vi "Image_processor.vi"(6 "DUT":u16, 9 "Ref Folder":path, 10 "DUT_Conf":string="RX-DUT", 11 "Image Path":path) -> (2 "Fail_Strings":string, 3 "PASS/FAIL":bool)   [LabVIEW 2025]
uses:
  Image_match_details.ctl
  <vilib>/Utility/file.llb/Read Delimited Spreadsheet (string).vi
panel:
  out "Array 3":T1[](array[typedef])
  out "Array 2":T1[](array[typedef])
  out "DUT":T2(plugin-control)
  out "Array":i32[](array[numeric])
  # "RY-DUT"
  # "RX-DUT"
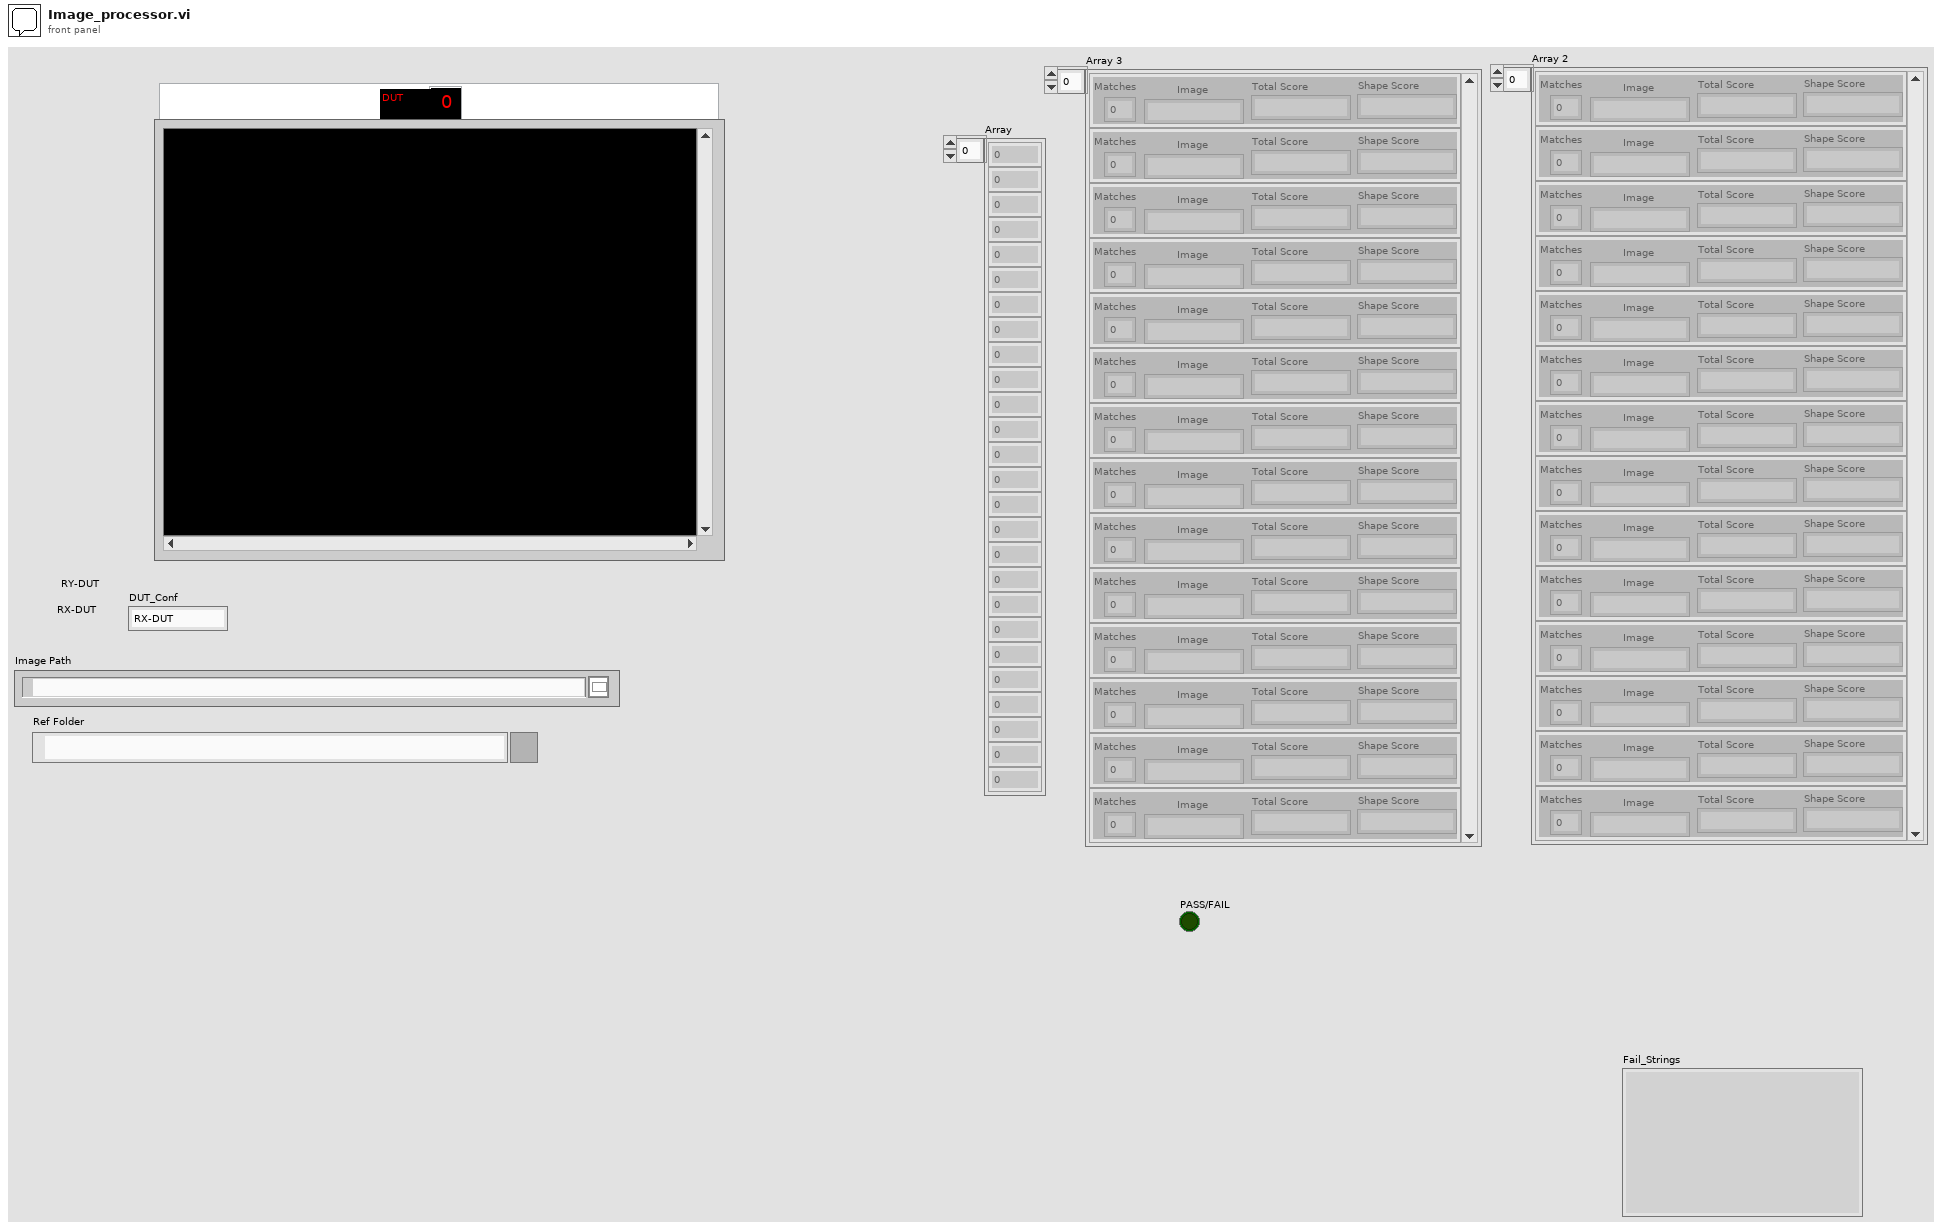
[diagram p1: front panel]
types:
  T1 = typedef "Image_match_details.ctl" = cluster{"Matches":i32, "Image":string, "Total Score":string, "Shape Score":string}
  T2 = typedef "IMAQ Image.ctl" = refnum<image>
  T3 = typedef "Image Type" = u32
  T4 = enum16{"open", "replace", "create", "open or create", "replace or create", "replace or create with confirmation"}
  T5 = cluster{"Position":cluster{"x":sgl, "y":sgl}, "Angle":sgl, "Scale":sgl, "Score":sgl, "Bounding Box":cluster{"x":sgl, "y":sgl}[]}
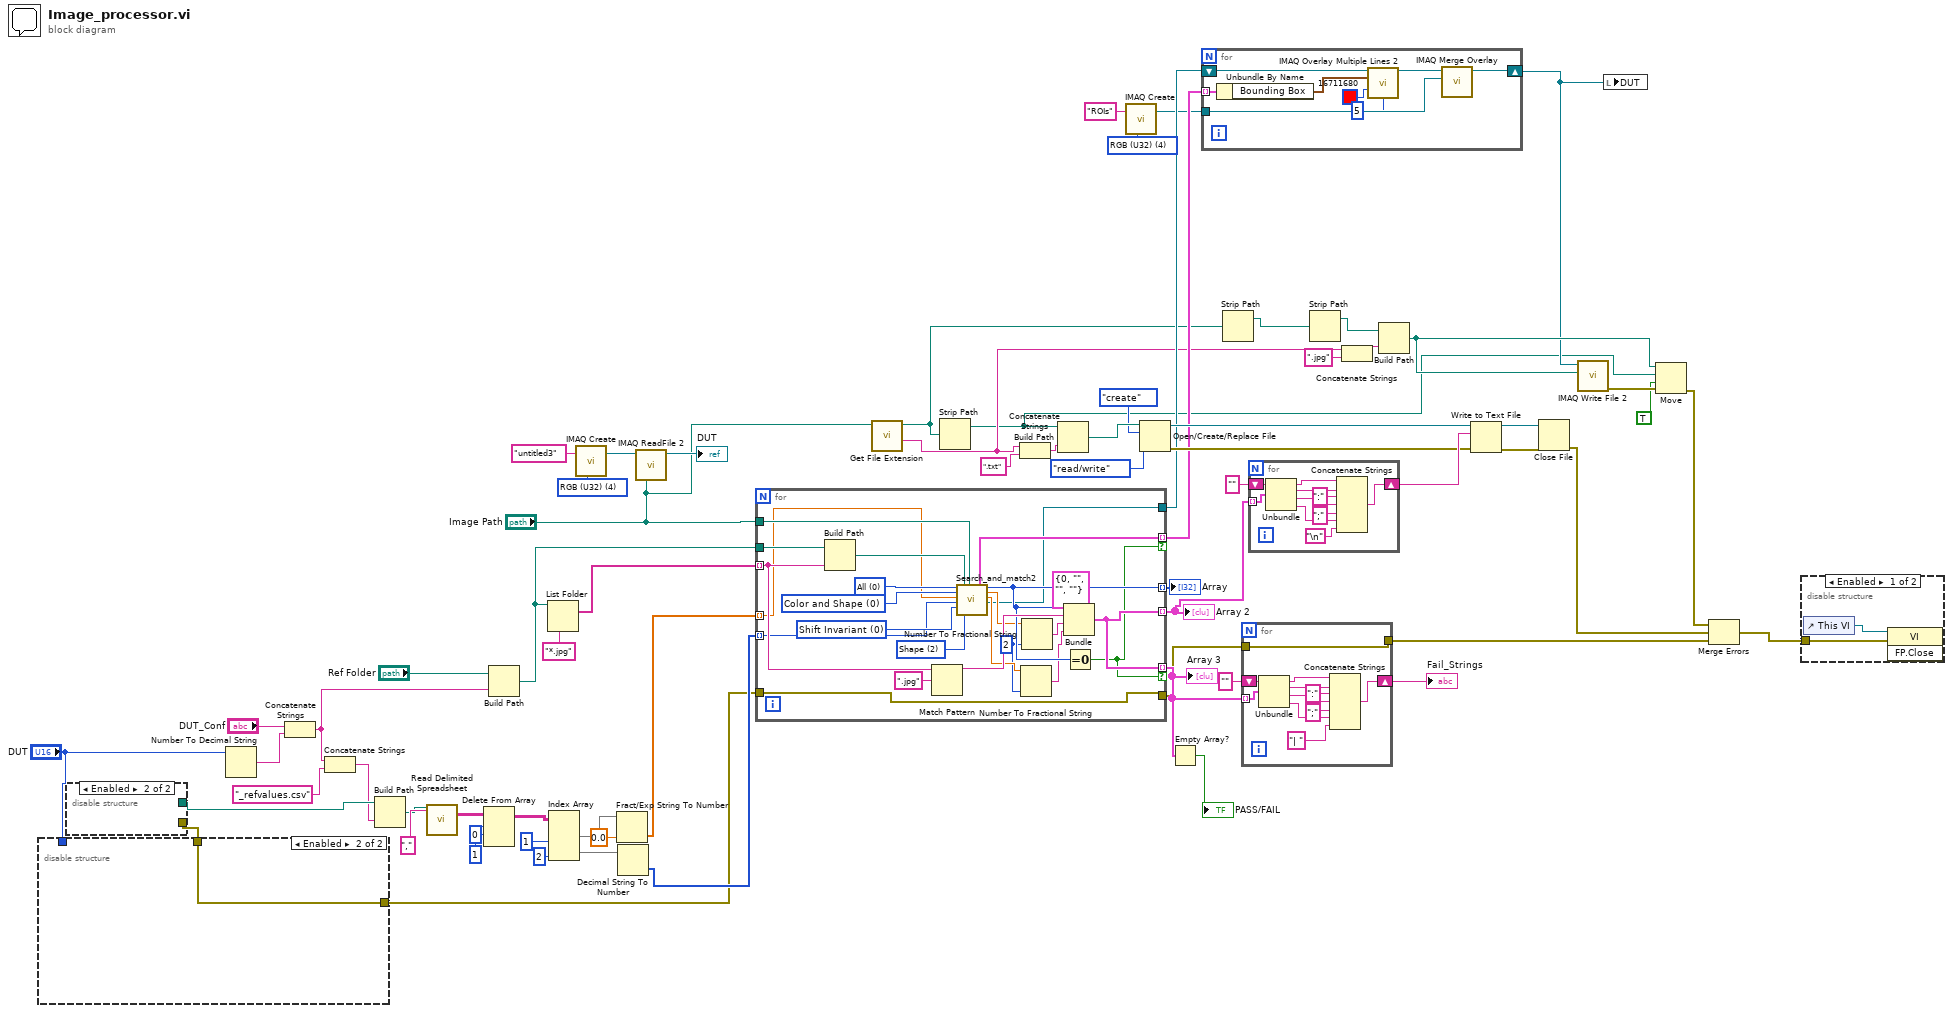
[diagram p0: block diagram]
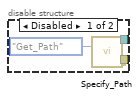
[diagram p2: hidden frame]
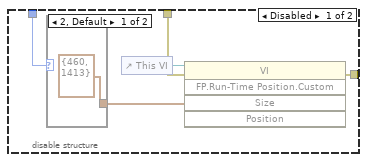
[diagram p3: hidden frame]
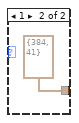
[diagram p4: hidden frame]
diagram:
  w17 = T3 4 items=["Grayscale (U8)", "Grayscale (I16)", "Grayscale (SGL)", "Complex (CSG)", "RGB (U32)", "HSL (U32)", "RGB (U64)", "Grayscale (U16)"] ("Image Type")
  w41 = T3 4 items=["Grayscale (U8)", "Grayscale (I16)", "Grayscale (SGL)", "Complex (CSG)", "RGB (U32)", "HSL (U32)", "RGB (U64)", "Grayscale (U16)"] ("Image Type")
  n1 = disable-structure shown="Enabled" {
    disable-tunnel: [w71 _] -> w51
    disable-tunnel: [w70 _] -> w37
    frame Disabled {
      n2 = call "Specify_Path.vi"("Path_Enum"=enum16{"Find_Path", "Get_Path"}."Get_Path") -> ("Configurations"=w71:path, "error out"=w70:errorcluster)  [unwired: 7 in, 6 out]
    }
    frame Enabled {
    }
  }
  n3 = disable-structure shown="Enabled" {
    disable-tunnel: w37 -> [w76 w80]
    disable-tunnel: "DUT" -> [w75 _]
    disable-tunnel: [w73 w80] -> w35
    frame Disabled {
      n4 = case shown="2, Default" w75 {
        tunnel: [cluster{"Top":i16, "Left":i16} {"Top"=460, "Left"=1413} ("Position") cluster{"Top":i16, "Left":i16} {"Top"=384, "Left"=41} ("Position")] -> w74
        frame 2, Default {
        }
        frame 1 {
        }
      }
      n5 = control-ref of="This VI"() -> (w77:refnum<vi>)
      n6 = invoke class="VI" method="FP.Run-Time Position.Custom"(reference=w77, error in=w76, "Size"=w74) -> (error out=w73:errorcluster)  [unwired: 2 in, 4 out]
    }
    frame Enabled {
    }
  }
  n7 = Number To Decimal String(number="DUT") -> (decimal integer string=w68:string)  [unwired: 1 in]
  n8 = Concatenate Strings("DUT_Conf", w68) -> (w53:string)
  n9 = Concatenate Strings(w53, "_refvalues.csv") -> (w50:string)
  n10 = Build Path(base path=w51, name or relative path=w50) -> (appended path=w49:path)
  n11 = call-poly <vilib>:"Read Delimited Spreadsheet.vi"("file path (dialog if empty)"=w49, "delimiter (\\t)"="," ("delimiter (\\t)")) -> ("all rows"=w61:string[][])  [unwired: 8 in, 5 out]
  n12 = Delete From Array(array=w61, length=1, index (row)=0) -> (array with subset deleted=w56:string[][])  [unwired: 1 in, 1 out]
  n13 = Build Path(base path="Ref Folder", name or relative path=w53) -> (appended path=w65:path)
  n14 = List Folder(path=w65, pattern="*.jpg") -> (filenames=w66:string[])  [unwired: 2 in, 3 out]
  n15 = Index Array(array=w56, index (col) #1=1 ("disabled index (col)"), index (col) #2=2 ("disabled index (col)")) -> (element #1=w58:string[], element #2=w57:string[])  [unwired: 2 in]
  n16 = call "IMAQ Create"("Image Name"="untitled3", "Image Type"=w41) -> ("New Image"=w39:T2)  [unwired: 3 in, 1 out]
  n17 = Fract/Exp String To Number(string=w58, default (0 dbl)=sgl 0.0 ("default (0 DBL)")) -> (number=w48:sgl[])  [unwired: 2 in, 1 out]
  n18 = Decimal String To Number(string=w57) -> (number=w47:i32[])  [unwired: 2 in, 1 out]
  n19 = call "IMAQ ReadFile 2"("File Path"="Image Path", "Image"=w39) -> ("Image Out"=→"DUT":T2)  [unwired: 5 in, 4 out]
  n20 = for {
    tunnel: w66 -> [w97] mode=indexing
    tunnel: w65 -> [w104]
    tunnel: "Image Path" -> [w102]
    tunnel: [w92] -> w64 mode=indexing
    tunnel: [w91] -> w32 mode=indexing
    tunnel: w48 -> [w94] mode=indexing
    tunnel: w47 -> [w93] mode=indexing
    tunnel: [w91] -> w43 mode=indexing if=w81
    tunnel: w35 -> [w88]
    tunnel: [w88] -> w34
    tunnel: [w83] -> w20 mode=indexing if=w81
    tunnel: [w82] -> w19
    w86 = i16 2 ("precision (6)")
    w98 = u32 2 items=["Color and Shape", "Color", "Shape"] ("Match Feature Mode")
    w99 = u32 0 items=["Shift Invariant", "Rotation Invariant"] ("Match Mode")
    w100 = u32 0 items=["Color and Shape", "Color", "Shape "] ("Feature Mode")
    w101 = u32 0 items=["All", "Shift Information", "Rotation Information"] ("Learn Mode")
    n21 = Build Path(base path=w104, name or relative path=w97) -> (appended path=w103:path)
    n22 = Match Pattern(string=w97, regular expression=".jpg") -> (before substring=w95:string)  [unwired: 1 in, 3 out]
    n23 = call "Search_and_match2.vi"("Learn Mode"=w101, "Feature Mode"=w100, "Minimum Match Score"=w94, "Number of Matches Requested"=w93, "Match Mode"=w99, "Ref path"=w103, "Match Feature Mode"=w98, "Main Path"=w102) -> ("Match values"=w83:T5, "Number of Matches"=w92:i32, "Total Score"=w90:sgl, "Shape Score"=w87:sgl, "Main Image"=w82:T2)  [unwired: 7 in]
    n24 = Number To Fractional String(number=w87, precision (6)=w86) -> (F-format string=w85:string)  [unwired: 2 in]
    n25 = Number To Fractional String(number=w90, precision (6)=w86) -> (F-format string=w89:string)  [unwired: 2 in]
    n26 = Bundle(cluster=T1 {"Matches"=0, "Image"="", "Total Score"="", "Shape Score"=""} ("output cluster"), "Matches"=w92, "Image"=w95, "Total Score"=w89, "Shape Score"=w85) -> (w91:T1)
    n27 = Equal To 0?(x=w92) -> (x = 0?=w81:bool)
  }
  "Array" <- w64
  "Array 2" <- w32
  "Array 3" <- w43
  n28 = call <vilib>:"Get File Extension.vi"("file"="Image Path") -> ("filename without extension"=w9:string, "dup file"=w12:path)  [unwired: 6 in, 3 out]
  n29 = Strip Path(path=w12) -> (stripped path=w4:path)  [unwired: 1 out]
  n30 = Concatenate Strings(w9, ".txt" ("string")) -> (w31:string)
  n31 = Build Path(base path=w4, name or relative path=w31) -> (appended path=w29:path)
  n32 = call "IMAQ Create"("Image Name"="ROIs", "Image Type"=w17) -> ("New Image"=w16:T2)  [unwired: 3 in, 1 out]
  n33 = Open/Create/Replace File(file path (use dialog)=w29, operation (0:open)=T4."create", access (0:read/write)=enum16{"read/write", "read-only", "write-only"}."read/write") -> (refnum out=w26:refnum<file>, error out=w25:errorcluster)  [unwired: 3 in, 1 out]
  n34 = Empty Array?(array=w43) -> (empty?=→"PASS/FAIL":bool)
  n35 = for {
    tunnel: w20 -> [w110] mode=indexing
    shift-right: [w107] -> w5
    shift-left: w19 -> [w112]
    tunnel: w16 -> [w106]
    n36 = Unbundle By Name(w110) -> ("Bounding Box"=w109:cluster{"x":sgl, "y":sgl}[])
    n37 = call "IMAQ Overlay Multiple Lines 2"("Image"=w112, "Line End Points"=w109, "Color"=u32 16711680, "Width"=u32 5) -> ("Image Out"=w108:T2)  [unwired: 10 in, 1 out]
    n38 = call "IMAQ Merge Overlay"("Image Dst"=w106, "Image Src"=w108) -> ("Image Dst Out"=w107:T2)  [unwired: 8 in, 1 out]
  }
  n39 = Strip Path(path=w12) -> (stripped path=w3:path)  [unwired: 1 out]
  n40 = for {
    tunnel: w43 -> [w122] mode=indexing
    shift-right: [w117] -> w44
    shift-left: "" -> [w116]
    tunnel: w34 -> [w115]
    tunnel: [w115] -> w33
    n41 = Unbundle(w122) -> ("Image"=w121:string, "Total Score"=w119:string, "Shape Score"=w113:string)  [unwired: 1 out]
    n42 = Concatenate Strings(w116, w121, ":" ("string"), w119, ";" ("string"), w113, "| " ("string")) -> (w117:string)
  }
  "Fail_Strings" <- w44
  n43 = for {
    tunnel: w32 -> [w131] mode=indexing
    shift-right: [w127] -> w27
    shift-left: "" -> [w126]
    n44 = Unbundle(w131) -> ("Image"=w130:string, "Total Score"=w128:string, "Shape Score"=w124:string)  [unwired: 1 out]
    n45 = Concatenate Strings(w126, w130, ":" ("string"), w128, ";" ("string"), w124, "\n") -> (w127:string)
  }
  n46 = Strip Path(path=w3) -> (stripped path=w11:path)  [unwired: 1 out]
  n47 = Concatenate Strings(w9, ".jpg" ("string")) -> (w10:string)
  n48 = Build Path(base path=w11, name or relative path=w10) -> (appended path=w6:path)
  n49 = Write to Text File(file (use dialog)=w26, text=w27, error in=w25) -> (refnum out=w22:refnum<file>, error out=w23:errorcluster)  [unwired: 1 in, 1 out]
  n50 = Close File(refnum=w22, error in=w23) -> (error out=w21:errorcluster)  [unwired: 1 out]
  n51 = call-poly "IMAQ Write File 2"("File Path"=w6, "Image"=w5) -> ("error out"=w15:errorcluster)  [unwired: 8 in, 1 out]
  n52 = local write "DUT"(w5) -> ()
  n53 = Move(source path=w6, error in=w15, 9:TRUE ("overwrite (F)"), 10:w4) -> (error out=w14:errorcluster)  [unwired: 1 in, 2 out]
  n54 = Merge Errors(w14, w21, w33) -> (w24:errorcluster)
  n55 = disable-structure shown="Enabled" {
    disable-tunnel: w24 -> [w132 _]
    frame Enabled {
      n56 = control-ref of="This VI"() -> (w133:refnum<vi>)
      n57 = invoke class="VI" method="FP.Close"(reference=w133, error in=w132) -> ()  [unwired: 1 in, 3 out]
    }
    frame Disabled {
    }
  }
